vi "DriveJoystickButtonMapping.vi"(11 "drive joystick buttons":bool[](array[boolean])) -> (3 "output cluster":T1, 4 "drive joystick buttons indicator":bool[](array[boolean]))   [LabVIEW 2018]
uses:
  Controls/DriveJoystickButtonMapping.ctl
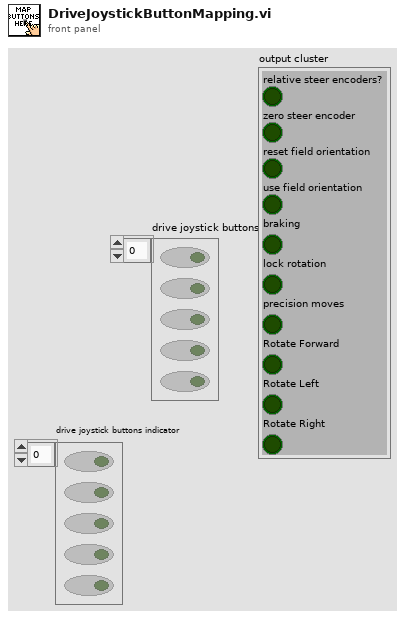
[diagram p1: front panel]
types:
  T1 = typedef "DriveJoystickButtonMapping.ctl" = cluster{"relative steer encoders?":bool, "zero steer encoder":bool, "reset field orientation":bool, "use field orientation":bool, "braking":bool, "lock rotation":bool, "precision moves":bool, "Rotate Forward":bool, "Rotate Left":bool, "Rotate Right":bool}
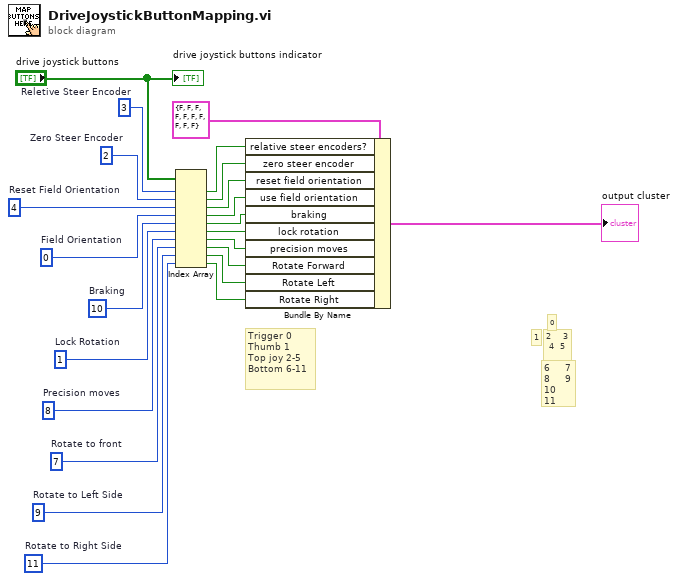
[diagram p0: block diagram]
diagram:
  w1 = 11  # Rotate to Right Side
  w2 = 9  # Rotate to Left Side
  w3 = 7  # Rotate to front
  w8 = 8  # Precision moves
  w9 = 1  # Lock Rotation
  w14 = 10  # Braking
  w20 = 0  # Field Orientation
  w21 = 4  # Reset Field Orientation
  w22 = 2  # Zero Steer Encoder
  w23 = 3  # Reletive Steer Encoder
  # "6     7\n8     9\n10  11"
  # "2    3\n 4  5"
  # "1"
  # "0"
  # "Trigger 0\nThumb 1\nTop joy 2-5\nBottom 6-11"
  n1 = Index Array(array="drive joystick buttons", index #1=w23, index #2=w22, index #3=w21, index #4=w20, index #5=w14, index #6=w9, index #7=w8, index #8=w3, index #9=w2, index #10=w1) -> (element #1=w18:bool, element #2=w17:bool, element #3=w16:bool, element #4=w15:bool, element #5=w13:bool, element #6=w12:bool, element #7=w7:bool, element #8=w6:bool, element #9=w5:bool, element #10=w4:bool)
  n2 = Bundle By Name(cluster=T1 {"relative steer encoders?"=FALSE, "zero steer encoder"=FALSE, "reset field orientation"=FALSE, "use field orientation"=FALSE, "braking"=FALSE, "lock rotation"=FALSE, "precision moves"=FALSE, "Rotate Forward"=FALSE, "Rotate Left"=FALSE, "Rotate Right"=FALSE} ("DriveJoystickButtonMapping"), "relative steer encoders?"=w18, "zero steer encoder"=w17, "reset field orientation"=w16, "use field orientation"=w15, "braking"=w13, "lock rotation"=w12, "precision moves"=w7, "Rotate Forward"=w6, "Rotate Left"=w5, "Rotate Right"=w4) -> (→"output cluster":T1)
  "drive joystick buttons indicator" <- "drive joystick buttons"
